vi "Sim and Debug.vi"(8 "error in":errorcluster, 11 "Path":path) -> (0 "error out":errorcluster, 1 "Debug?":bool, 2 "Development?":bool, 3 "Simulate?":bool)   [LabVIEW 2013]
doc: "This .vi checks to see if the files \"Simulate.txt\" , \"Development.txt\" (as opposed to Stable version), \"Debug.txt\" exist in the input path."
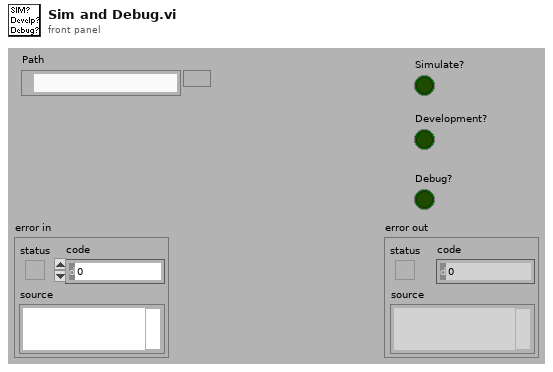
[diagram p1: front panel]
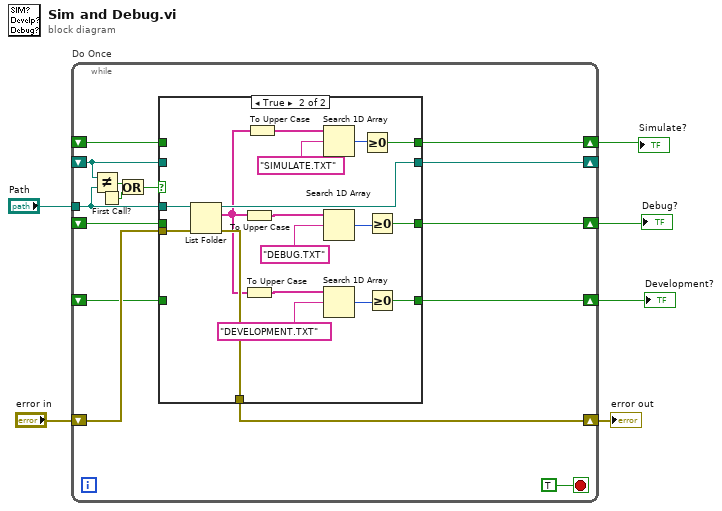
[diagram p0: block diagram]
diagram:
  n1 = while "Do Once" {
    tunnel: "Path" -> [w17]
    shift-right: [w18] -> w2
    shift-left: _ -> [w12]
    shift-right: [w19] -> w3
    shift-left: _ -> [w13]
    shift-right: [w11] -> _
    shift-left: _ -> [w10]
    shift-right: [w20] -> w4
    shift-left: "error in" -> [w21]
    shift-right: [w8] -> w1
    shift-left: _ -> [w7]
    stop <- TRUE stop-if-true
    n2 = Not Equal?(x=w10, y=w17) -> (x != y?=w15:bool)
    n3 = First Call?() -> (First Call?: T/F=w16:bool)
    n4 = Or(x=w15, y=w16) -> (x .or. y?=w14:bool)
    n5 = case shown="True" w14 {
      tunnel: w17 -> [_ w43]
      tunnel: w21 -> [w24 w42]
      tunnel: [w24 w41] -> w20
      tunnel: [w26 w34] -> w19
      tunnel: [w25 w33] -> w18
      tunnel: w13 -> [w26 _]
      tunnel: w12 -> [w25 _]
      tunnel: [w23 w32] -> w11
      tunnel: w10 -> [w23 _]
      tunnel: [w22 w27] -> w8
      tunnel: w7 -> [w22 _]
      frame False {
      }
      frame True {
        n6 = List Folder(path=w43, error in=w42) -> (path out=w32:path, filenames=w28:string[], error out=w41:errorcluster)  [unwired: 3 out]
        n7 = To Upper Case(1:w28) -> (0:w39:string[])
        n8 = To Upper Case(1:w28) -> (0:w30:string[])
        n9 = To Upper Case(1:w28) -> (0:w38:string[])
        n10 = Search 1D Array(1D array=w38, element="SIMULATE.TXT") -> (index of element=w36:i32)  [unwired: 1 out]
        n11 = Search 1D Array(1D array=w39, element="DEBUG.TXT") -> (index of element=w35:i32)  [unwired: 1 out]
        n12 = Search 1D Array(1D array=w30, element="DEVELOPMENT.TXT") -> (index of element=w31:i32)  [unwired: 1 out]
        n13 = Greater Or Equal To 0?(x=w36) -> (x >= 0?=w34:bool)
        n14 = Greater Or Equal To 0?(x=w35) -> (x >= 0?=w33:bool)
        n15 = Greater Or Equal To 0?(x=w31) -> (x >= 0?=w27:bool)
      }
    }
  }
  "error out" <- w4
  "Simulate?" <- w3
  "Debug?" <- w2
  "Development?" <- w1
